vi "MLUG_Provider_OnCommand.vi"(10 "Command ID":string, 11 "objects":T1[](array[typedef])) -> ()   [LabVIEW 2020]
uses:
  <resource>/Framework/Providers/API/ItemRef.ctl
panel:
  out "error out":errorcluster
  in  "error in":errorcluster
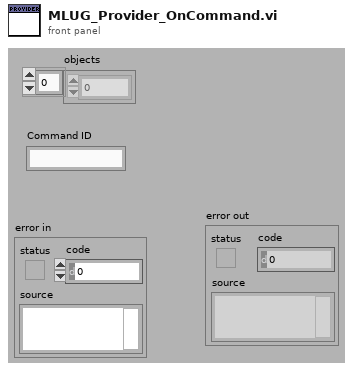
[diagram p1: front panel]
types:
  T1 = typedef "ItemRef.ctl" = u64
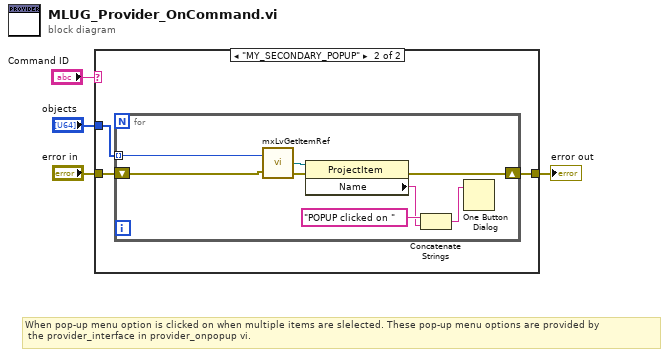
[diagram p0: block diagram]
diagram:
  # "When pop-up menu option is clicked on when multiple items are slelected. These pop-up menu options are provided by\n the provider_interface in provider_onpopup vi."
  n1 = case shown="\"MY_SECONDARY_POPUP\"" "Command ID" {
    tunnel: "objects" -> [_ w8]
    tunnel: "error in" -> [w5 w7]
    tunnel: [w5 w6] -> w1
    frame Default {
    }
    frame "MY_SECONDARY_POPUP" {
      n2 = for {
        tunnel: w8 -> [w16] mode=indexing
        shift-right: [w9] -> w6
        shift-left: w7 -> [w11]
        n3 = call <resource>:"mxLvGetItemRef.vi"("Item"=w16, "error in"=w11) -> ("Item Refnum"=w15:refnum<vi>, "error out"=w14:errorcluster)  [unwired: 1 out]
        n4 = property class="ProjectItem"(reference=w15, error in=w14) -> (error out=w9:errorcluster, "Name"=w12:string)  [unwired: 1 out]
        n5 = Concatenate Strings("POPUP clicked on " ("string"), w12) -> (w10:string)
        n6 = One Button Dialog(message=w10) -> ()  [unwired: 1 in, 1 out]
      }
    }
  }
  "error out" <- w1
